vi "CPMG_Pulse_CommandSTR_gen.vi"(0 "CPMG Pulse Sequence":T2={"Acquisition Settings"={"Number Samples"=2000, "Time Between Points"=0.0, "Unit"=0}, "Delay Settings"={"Delay d1"=10.0, "Delay d2"=0.0, "d1 Unit"=0, "d2 Unit"=0, "Delay d3"=0.0, "d3 Unit"=0, "Delay d4"=0.0, "d4 Unit"=0}, "Preliminary Settings"={"Nº of Scans (ns)"=3, "Pulse Frequency"=10000000.0, "Nº of Echoes (ne)"=3}, "Pulse Settings"={"Duration Signal P1"=20.0, "Power Level P1"=1023, "Phase P1"=90, "P1 Unit"=0, "Duration Signal P2"=20.0, "Power Level P2"=1023, "Phase P2"=90, "P2 Unit"=0}} {"Pulse Settings"."P2 Unit" items=["us", "ms"]; "Pulse Settings"."Phase P2" max=270 step=90; "Pulse Settings"."Power Level P2" max=1023 step=1; "Pulse Settings"."Duration Signal P2" min=0.0 step=1.0 format="%#_4g"; "Pulse Settings"."P1 Unit" items=["us", "ms"]; "Pulse Settings"."Phase P1" max=270 step=90; "Pulse Settings"."Power Level P1" max=1023 step=1; "Pulse Settings"."Duration Signal P1" min=0.0 step=1.0 format="%#_4g"; "Preliminary Settings"."Nº of Echoes (ne)" step=1; "Preliminary Settings"."Pulse Frequency" min=1.0 max=200000000.0 step=1000000.0 format="%^#_6e"; "Preliminary Settings"."Nº of Scans (ns)" step=1; "Delay Settings"."d4 Unit" items=["us", "ms"]; "Delay Settings"."Delay d4" min=0.0 step=1.0 format="%#_4g"; "Delay Settings"."d3 Unit" items=["us", "ms"]; "Delay Settings"."Delay d3" min=0.0 step=1.0 format="%#_4g"; "Delay Settings"."d2 Unit" items=["us", "ms"]; "Delay Settings"."d1 Unit" items=["us", "ms"]; "Delay Settings"."Delay d2" min=0.0 step=1.0 format="%#_4g"; "Delay Settings"."Delay d1" min=0.0 step=1.0 format="%#_4g"; "Acquisition Settings"."Unit" items=["us", "ms"]; "Acquisition Settings"."Time Between Points" min=0.0 step=1.0; "Acquisition Settings"."Number Samples" step=1}) -> (4 "CMD STR Array":string[](array[string]), 6 "CPMG Set Times":T1={"Real Time d4"=69.971913553241751126, "Real Time d3"=50.022661650188109273, "Real Time P2"=39.96053897978825603, "Real Time d2"=29.985913028261440076, "Real Time P1"=20.011287076734621636, "Real Time d1"=10.036661125207804438, "Real Time AQS"=0.73746299999999999998})   [LabVIEW 2011]
uses:
  Controls/Full_CPMG Degree Pulse Settings.ctl
  Controls/Acquisition Settings.ctl
  Controls/CPMG_Delay Settings.ctl
  Controls/CPMG_Preliminary Settings.ctl
  Controls/CPMG_Pulse Settings.ctl
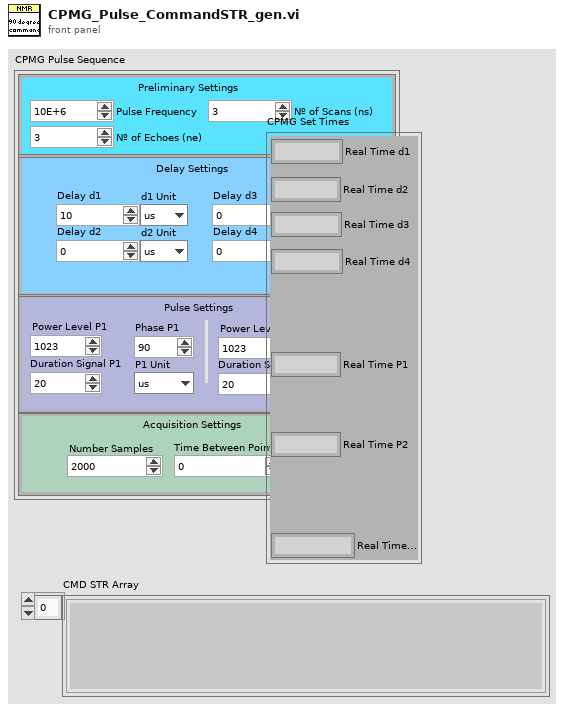
[diagram p1: front panel]
types:
  T1 = cluster{"Real Time d4":ext, "Real Time d3":ext, "Real Time P2":ext, "Real Time d2":ext, "Real Time P1":ext, "Real Time d1":ext, "Real Time AQS":ext}
  T2 = typedef "Full_CPMG Degree Pulse Settings.ctl" = cluster{"Acquisition Settings":T3, "Delay Settings":T4, "Preliminary Settings":T5, "Pulse Settings":T6}
  T3 = typedef "Acquisition Settings.ctl" = cluster{"Number Samples":u16, "Time Between Points":dbl, "Unit":u8}
  T4 = typedef "CPMG_Delay Settings.ctl" = cluster{"Delay d1":dbl, "Delay d2":dbl, "d1 Unit":u8, "d2 Unit":u8, "Delay d3":dbl, "d3 Unit":u8, "Delay d4":dbl, "d4 Unit":u8}
  T5 = typedef "CPMG_Preliminary Settings.ctl" = cluster{"Nº of Scans (ns)":u16, "Pulse Frequency":dbl, "Nº of Echoes (ne)":u16}
  T6 = typedef "CPMG_Pulse Settings.ctl" = cluster{"Duration Signal P1":dbl, "Power Level P1":u16, "Phase P1":u16, "P1 Unit":u8, "Duration Signal P2":dbl, "Power Level P2":u16, "Phase P2":u16, "P2 Unit":u8}
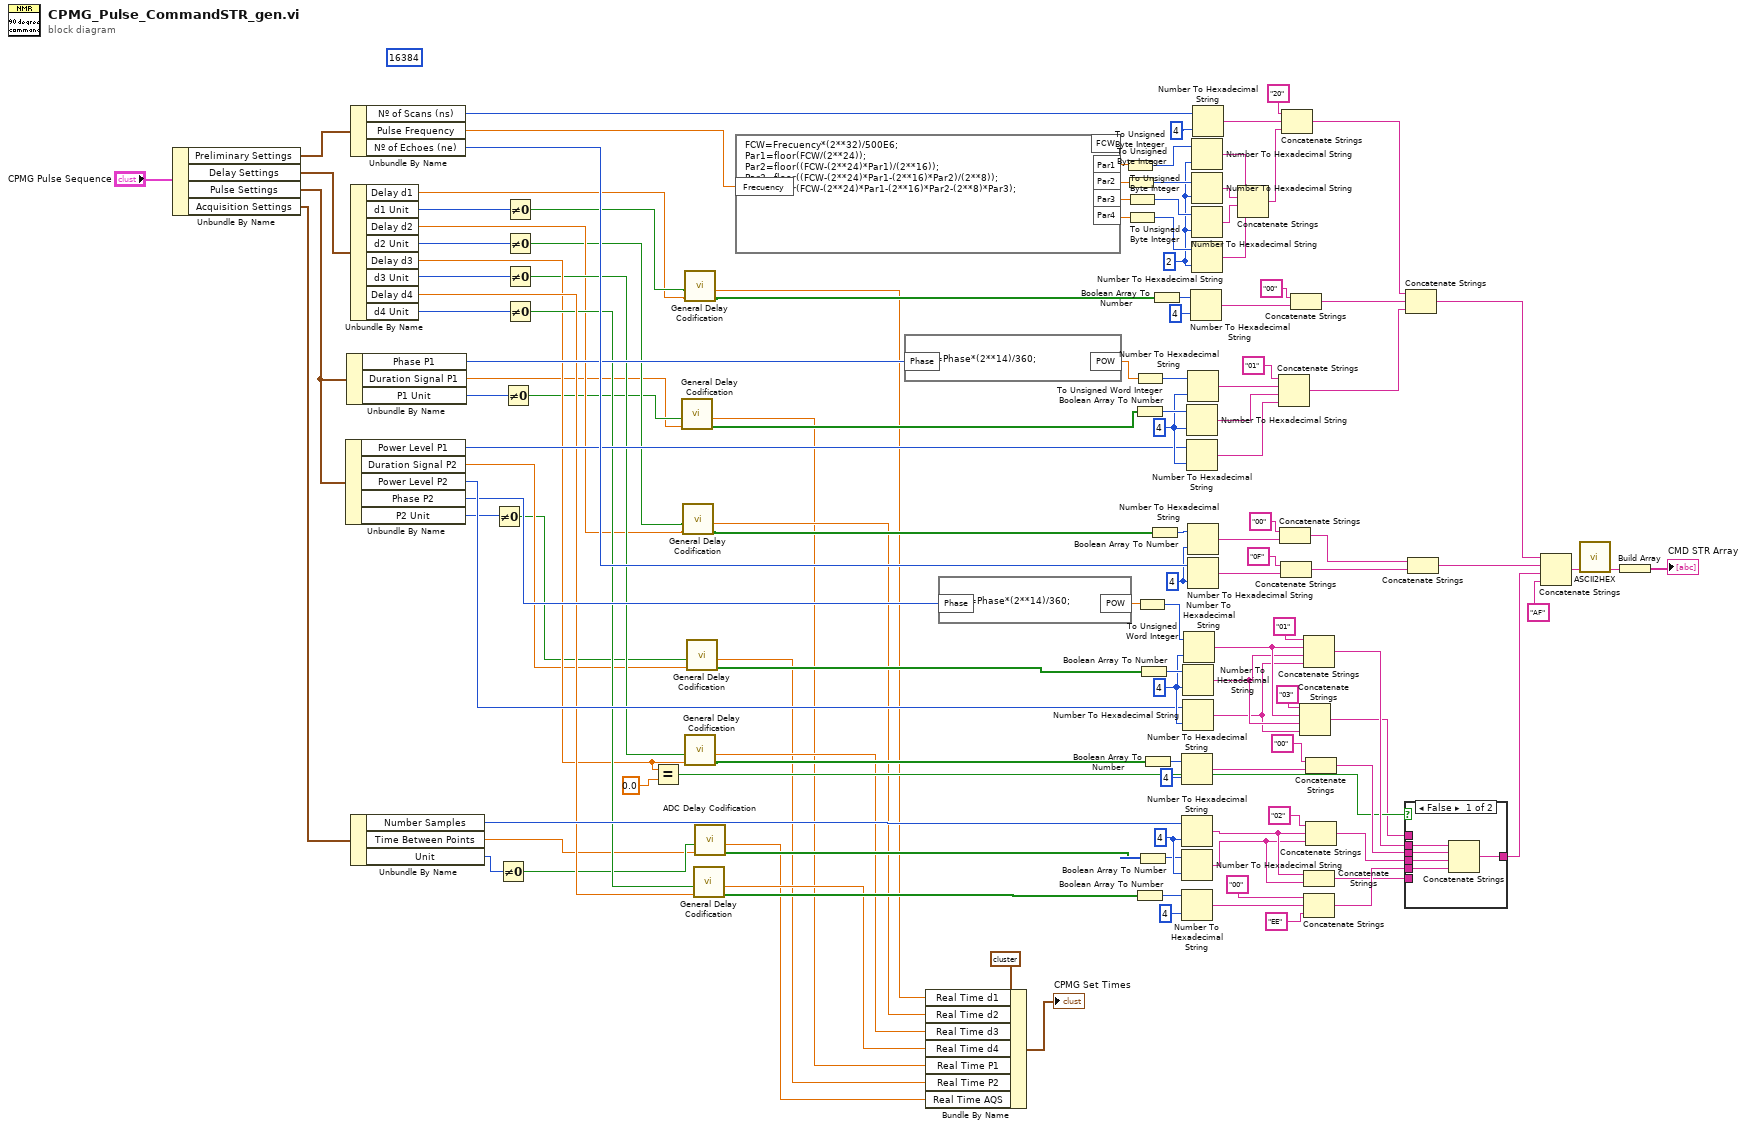
[diagram p0: block diagram]
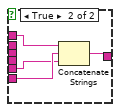
[diagram p2: hidden frame]
diagram:
  (unwired) u16 16384
  w73 = i16 2 ("width (-)")
  w108 = i16 4 ("width (-)")
  w48 = i16 4 ("width (-)")
  w36 = i16 4 ("width (-)")
  w49 = i16 4 ("width (-)")
  n1 = Unbundle By Name("CPMG Pulse Sequence") -> ("Preliminary Settings"=w128:T5, "Delay Settings"=w127:T4, "Pulse Settings"=w35:T6, "Acquisition Settings"=w126:T3)
  n2 = Unbundle By Name(w35) -> ("Power Level P1"=w42:u16, "Duration Signal P2"=w23:dbl, "Power Level P2"=w41:u16, "Phase P2"=w40:u16, "P2 Unit"=w39:u8)
  n3 = Unbundle By Name(w35) -> ("Phase P1"=w34:u16, "Duration Signal P1"=w16:dbl, "P1 Unit"=w33:u8)
  n4 = Unbundle By Name(w128) -> ("Nº of Scans (ns)"=w47:u16, "Pulse Frequency"=w46:dbl, "Nº of Echoes (ne)"=w45:u16)
  n5 = Unbundle By Name(w127) -> ("Delay d1"=w13:dbl, "d1 Unit"=w125:u8, "Delay d2"=w20:dbl, "d2 Unit"=w124:u8, "Delay d3"=w26:dbl, "d3 Unit"=w44:u8, "Delay d4"=w32:dbl, "d4 Unit"=w43:u8)
  n6 = Unbundle By Name(w126) -> ("Number Samples"=w38:u16, "Time Between Points"=w28:dbl, "Unit"=w123:u8)
  n7 = Not Equal To 0?(x=w39) -> (x != 0?=w22:bool)
  n8 = Not Equal To 0?(x=w123) -> (x != 0?=w29:bool)
  n9 = Not Equal To 0?(x=w33) -> (x != 0?=w17:bool)
  n10 = Not Equal To 0?(x=w125) -> (x != 0?=w14:bool)
  n11 = Not Equal To 0?(x=w124) -> (x != 0?=w19:bool)
  n12 = Not Equal To 0?(x=w44) -> (x != 0?=w25:bool)
  n13 = Not Equal To 0?(x=w43) -> (x != 0?=w31:bool)
  n14 = Equal?(x=w26, y=0.0) -> (x = y?=w58:bool)
  n15 = call "General Delay Codification.vi"("Delay"=w16, "ms/us Delay"=w17) -> ("Final array"=w15:bool[], "Real Time"=w3:ext)  [unwired: 8 in]
  n16 = call "General Delay Codification.vi"("Delay"=w20, "ms/us Delay"=w19) -> ("Final array"=w18:bool[], "Real Time"=w6:ext)  [unwired: 8 in]
  n17 = call "General Delay Codification.vi"("Delay"=w13, "ms/us Delay"=w14) -> ("Final array"=w12:bool[], "Real Time"=w7:ext)  [unwired: 8 in]
  n18 = call "General Delay Codification.vi"("Delay"=w26, "ms/us Delay"=w25) -> ("Final array"=w24:bool[], "Real Time"=w5:ext)  [unwired: 8 in]
  n19 = call "General Delay Codification.vi"("Delay"=w23, "ms/us Delay"=w22) -> ("Final array"=w21:bool[], "Real Time"=w2:ext)  [unwired: 8 in]
  n20 = call "General Delay Codification.vi"("Delay"=w32, "ms/us Delay"=w31) -> ("Final array"=w30:bool[], "Real Time"=w4:ext)  [unwired: 8 in]
  n21 = call "ADC Delay Codification.vi"("Delay"=w28, "ms/us Delay"=w29) -> ("Final array"=w27:bool[], "Real Time"=w1:ext)  [unwired: 8 in]
  n22 = formula code="FCW=Frecuency*(2**32)/500E6;\nPar1=floor(FCW/(2**24));\nPar2=floor((FCW-(2**24)*Par1)/(2**16));\nPar3=floor((FCW-(2**24)*Par1-(2**16)*Par2)/(2**8));\nPar4=floor(FCW-(2**24)*Par1-(2**16)*Par2-(2**8)*Par3);"("Frecuency"=w46) -> ("Par1"=w77:dbl, "Par2"=w76:dbl, "Par3"=w75:dbl, "Par4"=w74:dbl)  [unwired: 1 out]
  n23 = formula code="POW=Phase*(2**14)/360;"("Phase"=w34) -> ("POW"=w67:dbl)
  n24 = Bundle By Name(cluster=T1 {"Real Time d4"=69.971913553241751126, "Real Time d3"=50.022661650188109273, "Real Time P2"=39.96053897978825603, "Real Time d2"=29.985913028261440076, "Real Time P1"=20.011287076734621636, "Real Time d1"=10.036661125207804438, "Real Time AQS"=0.73746299999999999998} ("CPMG Set Times 2"), "Real Time d1"=w7, "Real Time d2"=w6, "Real Time d3"=w5, "Real Time d4"=w4, "Real Time P1"=w3, "Real Time P2"=w2, "Real Time AQS"=w1) -> (→"CPMG Set Times":T1)
  n25 = formula code="POW=Phase*(2**14)/360;"("Phase"=w40) -> ("POW"=w62:dbl)
  n26 = To Unsigned Byte Integer(number=w77) -> (unsigned 8bit integer=w81:u8)
  n27 = To Unsigned Byte Integer(number=w76) -> (unsigned 8bit integer=w80:u8)
  n28 = To Unsigned Byte Integer(number=w75) -> (unsigned 8bit integer=w79:u8)
  n29 = To Unsigned Byte Integer(number=w74) -> (unsigned 8bit integer=w78:u8)
  n30 = To Unsigned Word Integer(number=w67) -> (unsigned 16bit integer=w66:u16)
  n31 = Boolean Array To Number(Boolean array=w15) -> (number=w88:u32)
  n32 = Boolean Array To Number(Boolean array=w30) -> (number=w84:u32)
  n33 = To Unsigned Word Integer(number=w62) -> (unsigned 16bit integer=w61:u16)
  n34 = Boolean Array To Number(Boolean array=w27) -> (number=w83:u32)
  n35 = Boolean Array To Number(Boolean array=w21) -> (number=w85:u32)
  n36 = Boolean Array To Number(Boolean array=w24) -> (number=w86:u32)
  n37 = Boolean Array To Number(Boolean array=w18) -> (number=w87:u32)
  n38 = Boolean Array To Number(Boolean array=w12) -> (number=w89:u32)
  n39 = Number To Hexadecimal String(1:i16 4 ("width (-)"), 2:w86) -> (0:w110:string)
  n40 = Number To Hexadecimal String(1:w108, 2:w38) -> (0:w53:string)
  n41 = Number To Hexadecimal String(1:w108, 2:w83) -> (0:w52:string)
  n42 = Number To Hexadecimal String(1:i16 4 ("width (-)"), 2:w84) -> (0:w105:string)
  n43 = Number To Hexadecimal String(1:w48, 2:w85) -> (0:w55:string)
  n44 = Number To Hexadecimal String(1:w48, 2:w41) -> (0:w54:string)
  n45 = Number To Hexadecimal String(1:w48, 2:w61) -> (0:w56:string)
  n46 = Number To Hexadecimal String(1:w49, 2:w88) -> (0:w64:string)
  n47 = Number To Hexadecimal String(1:w49, 2:w42) -> (0:w63:string)
  n48 = Number To Hexadecimal String(1:w49, 2:w66) -> (0:w65:string)
  n49 = Number To Hexadecimal String(1:w36, 2:w87) -> (0:w116:string)
  n50 = Number To Hexadecimal String(1:w36, 2:w45) -> (0:w114:string)
  n51 = Number To Hexadecimal String(1:i16 4 ("width (-)"), 2:w89) -> (0:w119:string)
  n52 = Number To Hexadecimal String(1:w73, 2:w81) -> (0:w72:string)
  n53 = Number To Hexadecimal String(1:w73, 2:w80) -> (0:w71:string)
  n54 = Number To Hexadecimal String(1:w73, 2:w79) -> (0:w70:string)
  n55 = Number To Hexadecimal String(1:w73, 2:w78) -> (0:w69:string)
  n56 = Number To Hexadecimal String(1:i16 4 ("width (-)"), 2:w47) -> (0:w102:string)
  n57 = Concatenate Strings(w72, w71, w70, w69) -> (w68:string)
  n58 = Concatenate Strings("01" ("string"), w65, w64, w63) -> (w98:string)
  n59 = Concatenate Strings("00" ("string"), w116) -> (w97:string)
  n60 = Concatenate Strings("0F" ("string"), w114) -> (w96:string)
  n61 = Concatenate Strings("20" ("string"), w102, w68) -> (w100:string)
  n62 = Concatenate Strings("00" ("string"), w119) -> (w99:string)
  n63 = Concatenate Strings("03" ("string"), w56, w55, w54) -> (w51:string)
  n64 = Concatenate Strings("01" ("string"), w56, w55, w54) -> (w60:string)
  n65 = Concatenate Strings(w53, w52) -> (w50:string)
  n66 = Concatenate Strings("00" ("string"), w105, "EE" ("string")) -> (w93:string)
  n67 = Concatenate Strings("00" ("string"), w110) -> (w95:string)
  n68 = Concatenate Strings("02" ("string"), w53, w52) -> (w94:string)
  n69 = case shown="False" w58 {
    tunnel: w95 -> [w133 _]
    tunnel: w94 -> [w132 _]
    tunnel: w93 -> [w131 w134]
    tunnel: [w130 w137] -> w92
    tunnel: w60 -> [w129 _]
    tunnel: w51 -> [_ w136]
    tunnel: w50 -> [_ w135]
    frame False {
      n70 = Concatenate Strings(w129, w133, w132, w131) -> (w130:string)
    }
    frame True {
      n71 = Concatenate Strings(w136, w135, w134) -> (w137:string)
    }
  }
  n72 = Concatenate Strings(w100, w99, w98) -> (w90:string)
  n73 = Concatenate Strings(w97, w96) -> (w91:string)
  n74 = Concatenate Strings(w90, w91, w92, "AF" ("string")) -> (w37:string)
  n75 = call "ASCII2HEX.vi"("String (Normal Display)"=w37) -> ("Result string (Hex Display)"=w11:string)  [unwired: 10 in]
  n76 = Build Array(w11) -> (→"CMD STR Array":string[])
